vi "Get Table Column Values (VAR).vi"(7 "Sheet Name in":string, 8 "error in":errorcluster, 9 "Column Name":string, 10 "Table Name":string, 11 "SpreadsheetDoc in":refnum<k24>) -> (0 "error out":errorcluster, 2 "Column Values":variant[](array[variant]), 3 "SpreadsheetDoc out":refnum<k24>, 5 "Sheet Name out":string)   [LabVIEW 2019, in "Open Xml.lvlib"]
uses:
  Open Xml.lvlib
  D:/git/Open-Xml-LabVIEW/Source/DocumentFormat.OpenXml.dll
  DocumentFormat.OpenXml.dll
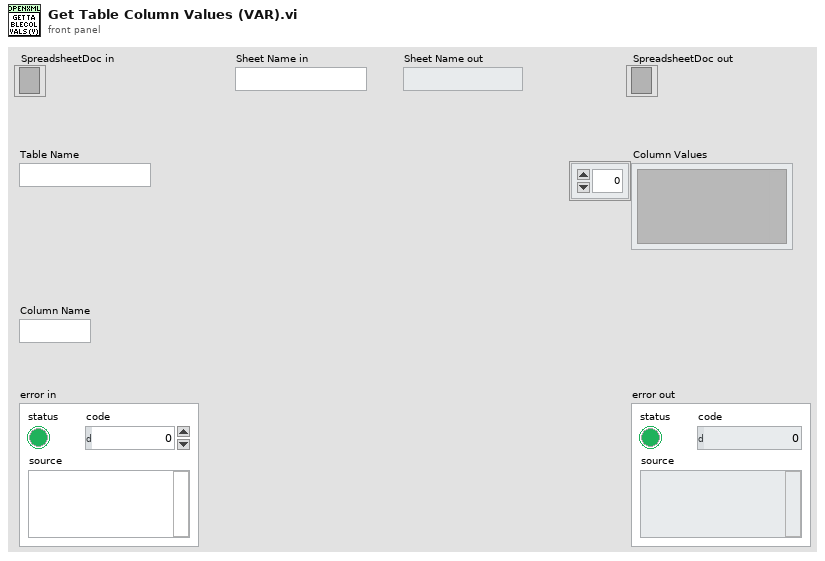
[diagram p1: front panel]
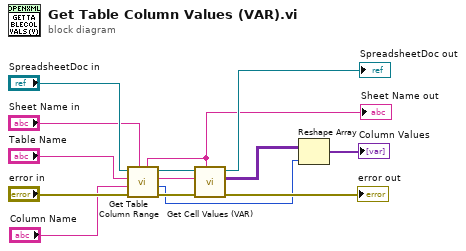
[diagram p0: block diagram]
diagram:
  n1 = call "Get Table Column Range.vi"("Sheet Name in"="Sheet Name in", "error in"="error in", "Column Name"="Column Name", "Table Name"="Table Name", "SpreadsheetDoc in"="SpreadsheetDoc in") -> ("error out"=w12:errorcluster, "Row Count"=w4:i32, "Range"=w3:string, "SpreadsheetDoc out"=w10:refnum<k24>, "Sheet Name out"=w1:string)  [unwired: 2 in]
  "Sheet Name out" <- w1
  n2 = call "Get Cell Values (VAR).vi"("Sheet Name in"=w1, "error in"=w12, "Cell Range"=w3, "SpreadsheetDoc in"=w10) -> ("error out"=→"error out":errorcluster, "Cell Values"=w8:variant[][], "SpreadsheetDoc out"=→"SpreadsheetDoc out":refnum<k24>)  [unwired: 5 in]
  n3 = Reshape Array(w8, w4) -> (→"Column Values":variant[])
